vi "UIRef.vi"(8 "error in":errorcluster, 11 "CVS in":refnum<class "PLTarget CVS.lvclass">) -> (0 "error out":errorcluster, 2 "VI refnum":refnum<vi>, 3 "CVS out":refnum<class "PLTarget CVS.lvclass">)   [LabVIEW 2013, in "PLTarget CVS.lvclass"]
uses:
  PLTarget CVS.lvclass
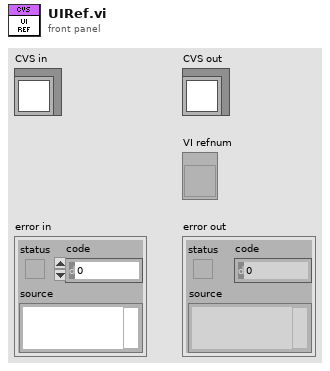
[diagram p1: front panel]
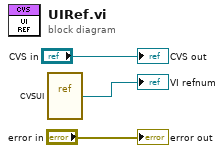
[diagram p0: block diagram]
diagram:
  n1 = vi-ref "CVSUI.vi"() -> (→"VI refnum":refnum<vi>)
  "error out" <- "error in"
  "CVS out" <- "CVS in"
